vi "serialiseArray.vi"(11 "GraphPeripherals":T1[][](array[typedef])) -> (3 "output array":T1[](array[typedef]))   [LabVIEW 2012]
uses:
  graphPeripherals.ctl
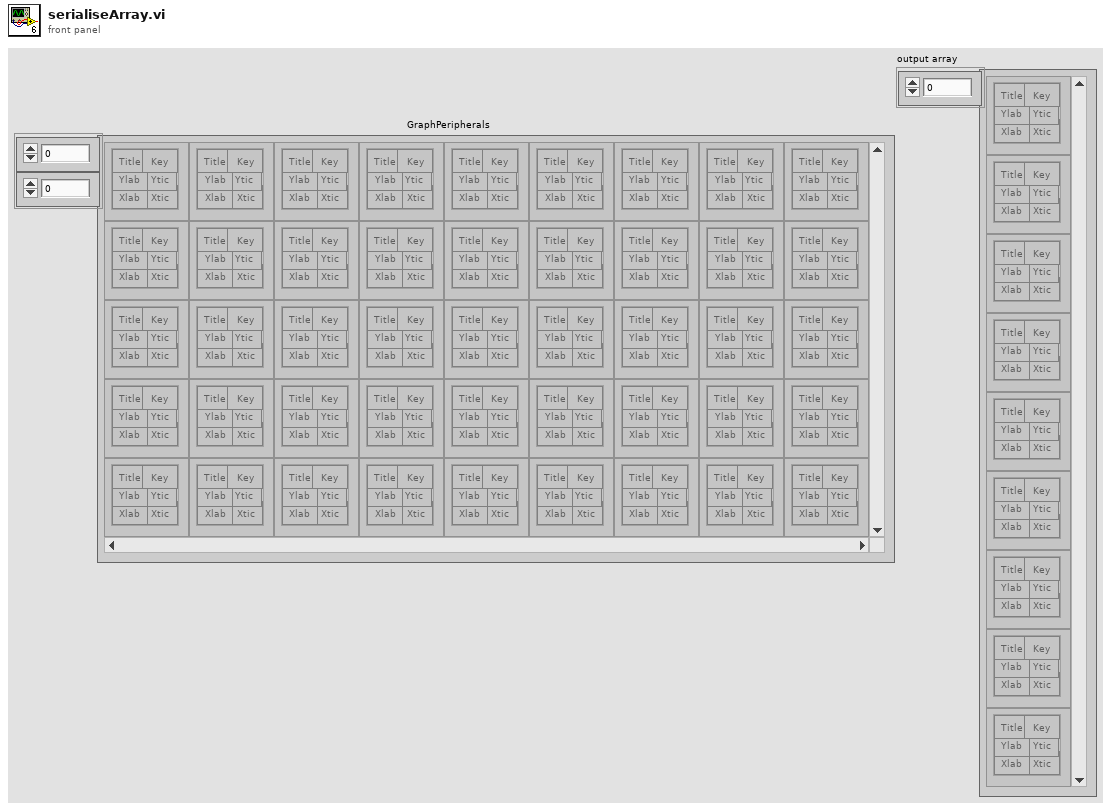
[diagram p1: front panel]
types:
  T1 = typedef "graphPeripherals.ctl" = cluster{"title":bool, "key":bool, "Xtic":bool, "Ytic":bool, "Xlab":bool, "Ylab":bool}
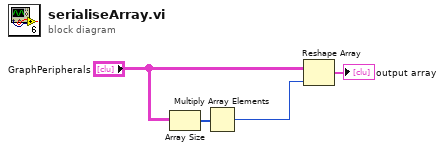
[diagram p0: block diagram]
diagram:
  n1 = Array Size(array="GraphPeripherals") -> (size(s)=w2:i32[])
  n2 = Multiply Array Elements(1:w2) -> (0:w1:i32)
  n3 = Reshape Array("GraphPeripherals", w1) -> (→"output array":T1[])
